vi "plugin test.vi"() -> ()   [LabVIEW 2013, in "CLFN tests.lvlib"]
uses:
  CLFN tests.lvlib
  execution/Shared Library Module runtime.lvclass
  configuration/Shared Library Module configuration.lvclass
  configuration/Shared Library Module configuration.lvclass/Shared Library Module configuration.ctl
  <vilib>/NI/Tag Bus Module Framework/channel/channel classification.ctl
  <vilib>/NI/Tag Bus/table/data polymorphs/write one/write Double.vi
  <vilib>/NI/Tag Bus/table/data polymorphs/write one/write Single.vi
  <vilib>/NI/Tag Bus/table/data polymorphs/read one/read Double.vi
  <vilib>/NI/Tag Bus/table/data polymorphs/read one/read Single.vi
  configuration/Write dllpath.vi
  <vilib>/NI/Tag Bus Module Framework/channel/TBM channel.lvclass
  <vilib>/NI/Tag Bus/dictionary/data dictionary.lvclass
  <vilib>/NI/Tag Bus/table/data table.lvlib
panel:
  out "final error":errorcluster
  out "result lookup err":errorcluster
  out "func error":errorcluster
  out "param lookup error":errorcluster
  out "result":dbl[](array[numeric])
  in  "parameter":dbl[](array[numeric])=[3.0, 5.0]
  out "correct exec settings":bool
  out "serialization error":errorcluster
  out "cfg error":errorcluster
  out "operation error":errorcluster
  out "header error":errorcluster
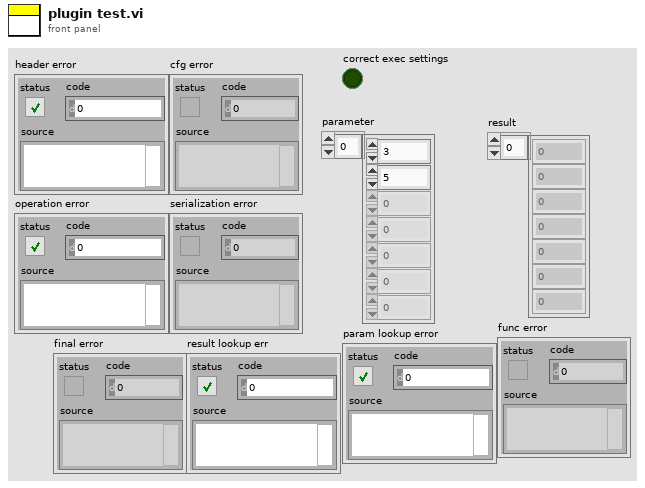
[diagram p1: front panel]
types:
  T1 = typedef "TBM channel.lvclass/channel classification.ctl" = enum16{"input data", "output data", "processing parameter", "processing result"}
  T2 = typedef "tag bus.lvlib/tag descriptor.lvclass/Data Type.ctl" = enum16{"Double", "Single", "I64", "I32", "I16", "I8", "U64", "U32", "U16", "U8", "Boolean", "String", "Array of Double", "Array of Single", "Array of I64", "Array of I32", "Array of I16", "Array of I8", "Array of U64", "Array of U32", "Array of U16", "Array of U8", "Array of Boolean", "Array of String"}
  T3 = typedef "TBM channel.lvclass/data tables.ctl" = cluster{"input data":T4, "processing parameter":T4, "processing result":T4, "output data":T4}
  T4 = typedef "tag bus.lvlib/dictionary table pair.ctl" = cluster{"data dictionary":refnum<class "data dictionary.lvclass">, "data table":T5}
  T5 = typedef "tag bus.lvlib/data table.lvlib/data table.ctl" = cluster{"Double":dbl[], "Single":sgl[], "I64":i64[], "I32":i32[], "I16":i16[], "I8":i8[], "U64":u64[], "U32":u32[], "U16":u16[], "U8":u8[], "Boolean":bool[], "String":string[], "Array of Double":cluster{"DBL Array":dbl[]}[], "Array of Single":cluster{"SGL Array":sgl[]}[], "Array of I64":cluster{"I64 Array":i64[]}[], "Array of I32":cluster{"I32 Array":i32[]}[], "Array of I16":cluster{"I16 Array":i16[]}[], "Array of I8":cluster{"I8 Array":i8[]}[], "Array of U64":cluster{"U64 Array":u64[]}[], "Array of U32":cluster{"U32 Array":u32[]}[], "Array of U16":cluster{"U16 Array":u16[]}[], "Array of U8":cluster{"U8 Array":u8[]}[], "Array of Boolean":cluster{"Boolean Array":bool[]}[], "Array of String":cluster{"String Array":string[]}[]}
  T6 = typedef "TBM module execution interface.lvclass/execution settings.ctl" = cluster{"reads inputs":bool, "processes data":bool, "writes outputs":bool}
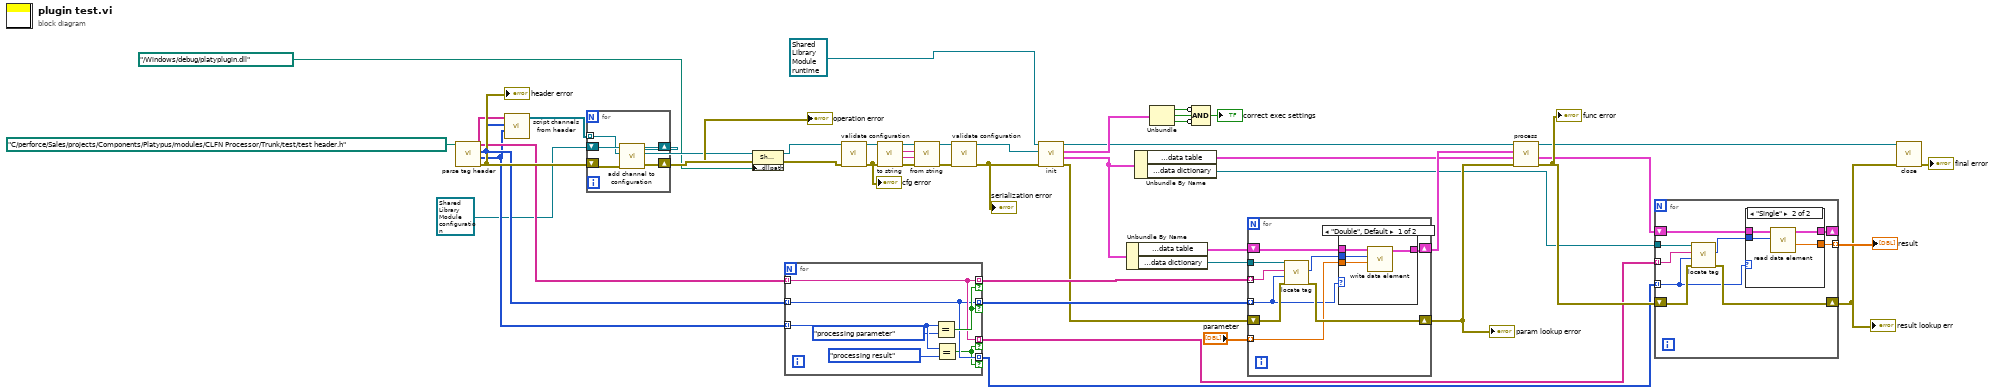
[diagram p0: block diagram]
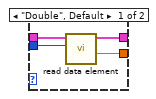
[diagram p2: hidden frame]
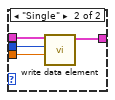
[diagram p3: hidden frame]
diagram:
  n1 = call "parse tag header.vi"("Path"=path "C:/perforce/Sales/projects/Components/Platypus/modules/CLFN Processor/Trunk/test/test header.h") -> ("error out"=w47:errorcluster, "classifications"=w27:T1[], "types"=w28:T2[], "names"=w29:string[])  [unwired: 7 in]
  "header error" <- w47
  n2 = call "script channels from header.vi"("classifications"=w27, "types"=w28, "names"=w29) -> ("channels"=w46:refnum<class "TBM channel.lvclass">[])  [unwired: 8 in]
  n3 = for {
    shift-right: [w53] -> w5
    shift-left: refnum<class "Shared Library Module configuration.lvclass"> refnum ("Shared Library Module configuration") -> [w50]
    tunnel: w46 -> [w49] mode=indexing
    shift-right: [w52] -> w45
    shift-left: w47 -> [w51]
    n4 = call "add channel to configuration.vi"("error in"=w51, "TBM channel in"=w49, "Shared Library Module configuration in"=w50) -> ("error out"=w52:errorcluster, "Shared Library Module configuration out"=w53:refnum<class "Shared Library Module configuration.lvclass">)  [unwired: 7 in]
  }
  n5 = property class="Shared Library Module configura"(reference=w5, error in=w45, "data access:dllpath"=path "../Windows/debug/platyplugin.dll" ("Path")) -> (reference out=w4:refnum<class "Shared Library Module configuration.lvclass">, error out=w6:errorcluster)
  "operation error" <- w6
  n6 = for {
    tunnel: w29 -> [w56] mode=indexing
    tunnel: w28 -> [w55] mode=indexing
    tunnel: w27 -> [w60] mode=indexing
    tunnel: [w56] -> w26 mode=indexing if=w57
    tunnel: [w55] -> w25 mode=indexing if=w57
    tunnel: [w56] -> w12 mode=indexing if=w54
    tunnel: [w55] -> w11 mode=indexing if=w54
    n7 = Equal?(x=w60, y=channel_classification."processing parameter") -> (x = y?=w57:bool)
    n8 = Equal?(x=w60, y=channel_classification."processing result") -> (x = y?=w54:bool)
  }
  n9 = call-dynamic "validate configuration.vi"("error in"=w6, "Shared Library Module configuration in"=w4) -> ("error out"=w44:errorcluster, "Shared Library Module configuration out"=w43:refnum<class "Shared Library Module configuration.lvclass">)  [unwired: 8 in]
  "cfg error" <- w44
  n10 = call-dynamic "to string.vi"("error in"=w44, "Shared Library Module configuration in"=w43) -> ("error out"=w41:errorcluster, "data"=w40:string, "version"=w39:string, "Shared Library Module configuration out"=w42:refnum<class "Shared Library Module configuration.lvclass">)  [unwired: 6 in]
  n11 = call-dynamic "from string.vi"("error in"=w41, "data"=w40, "version"=w39, "Shared Library Module configuration in"=w42) -> ("error out"=w37:errorcluster, "Shared Library Module configuration out"=w38:refnum<class "Shared Library Module configuration.lvclass">)  [unwired: 6 in]
  n12 = call-dynamic "validate configuration.vi"("error in"=w37, "Shared Library Module configuration in"=w38) -> ("error out"=w36:errorcluster, "Shared Library Module configuration out"=w35:refnum<class "Shared Library Module configuration.lvclass">)  [unwired: 8 in]
  "serialization error" <- w36
  n13 = call-dynamic "init.vi"("error in"=w36, "TBM module configuration in"=w35, "Shared Library Module runtime in"=refnum<class "Shared Library Module runtime.lvclass"> refnum ("Shared Library Module runtime")) -> ("error out"=w22:errorcluster, "data allocations"=w18:T3, "execution settings"=w34:T6, "Shared Library Module runtime out"=w16:refnum<class "Shared Library Module runtime.lvclass">)  [unwired: 5 in]
  n14 = Unbundle By Name(w18) -> ("processing parameter.data table"=w24:T5, "processing parameter.data dictionary"=w23:refnum<class "data dictionary.lvclass">)
  n15 = Unbundle By Name(w18) -> ("processing result.data table"=w17:T5, "processing result.data dictionary"=w13:refnum<class "data dictionary.lvclass">)
  n16 = Unbundle(w34) -> ("reads inputs"=w31:bool, "processes data"=w32:bool, "writes outputs"=w33:bool)
  n17 = Compound Arithmetic op=AND(invert w31, w32, invert w33) -> (→"correct exec settings":bool)
  n18 = for {
    tunnel: w26 -> [w67] mode=indexing
    tunnel: w25 -> [w61] mode=indexing
    shift-right: [w64] -> w19
    shift-left: w24 -> [w65]
    tunnel: w23 -> [w69]
    shift-right: [w66] -> w20
    shift-left: w22 -> [w68]
    tunnel: "parameter" -> [w62] mode=indexing
    n19 = call <vilib>:"locate tag.vi"("error in"=w68, "data type"=w61, "name"=w67, "data dictionary in"=w69) -> ("error out"=w66:errorcluster, "index"=w63:i32)  [unwired: 5 in, 1 out]
    n20 = case shown="\"Double\", Default" w61 {
      tunnel: w65 -> [w73 w77]
      tunnel: [w72 w76] -> w64
      tunnel: w63 -> [w71 w75]
      tunnel: w62 -> [w70 w74]
      frame "Double", Default {
        n21 = call-poly <vilib>:"write data element.vi"("value"=w70, "index"=w71, "data table in"=w73) -> ("data table out"=w72:T5)  [unwired: 8 in]
      }
      frame "Single" {
        n22 = call-poly <vilib>:"write data element.vi"("value"=w74, "index"=w75, "data table in"=w77) -> ("data table out"=w76:T5)  [unwired: 8 in]
      }
    }
  }
  "param lookup error" <- w20
  n23 = call-dynamic "process.vi"("error in"=w20, "result allocation"=w17, "parameters"=w19, "module in"=w16) -> ("error out"=w15:errorcluster, "results"=w14:T5, "module out"=w9:refnum<class "Shared Library Module runtime.lvclass">)  [unwired: 4 in, 1 out]
  "func error" <- w15
  n24 = for {
    tunnel: w12 -> [w84] mode=indexing
    tunnel: w11 -> [w79] mode=indexing
    shift-right: [w81] -> _
    shift-left: w14 -> [w82]
    tunnel: w13 -> [w86]
    shift-right: [w83] -> w8
    shift-left: w15 -> [w85]
    tunnel: [w78] -> w10 mode=indexing
    n25 = call <vilib>:"locate tag.vi"("error in"=w85, "data type"=w79, "name"=w84, "data dictionary in"=w86) -> ("error out"=w83:errorcluster, "index"=w80:i32)  [unwired: 5 in, 1 out]
    n26 = case shown="\"Single\"" w79 {
      tunnel: w82 -> [w89 w94]
      tunnel: [w90 w93] -> w81
      tunnel: w80 -> [w88 w92]
      tunnel: [w87 w91] -> w78
      frame "Double", Default {
        n27 = call-poly <vilib>:"read data element.vi"("index"=w88, "data table in"=w89) -> ("value"=w87:dbl, "data table out"=w90:T5)  [unwired: 8 in]
      }
      frame "Single" {
        n28 = call-poly <vilib>:"read data element.vi"("index"=w92, "data table in"=w94) -> ("value"=w91:sgl, "data table out"=w93:T5)  [unwired: 8 in]
      }
    }
  }
  "result" <- w10
  "result lookup err" <- w8
  n29 = call-dynamic "close.vi"("error in"=w8, "Shared Library Module runtime in"=w9) -> ("error out"=→"final error":errorcluster)  [unwired: 9 in]
